vi "Pickering 4 wire.vi"(0 "26":string[](array[combo])=["y5"], 1 "27":string[](array[combo])=["NC"], 2 "28":string[](array[combo])=["y3"], 3 "1":string[](array[combo])=["y4", "NC"], 8 "5":string[](array[combo])=["NC"], 9 "4":string[](array[combo])=["y6"], 10 "3":string[](array[combo])=["NC"], 11 "2":string[](array[combo])=["y1"]) -> ()   [LabVIEW 2011]
panel:
  in  "Initialize":bool
  in  "Pickering status":path=path "C:/LabView/PPMS basic VIs/Switch Status.txt"
  in  "Disconnect all?":bool
  in  "IVI Option String":string="Simulate=0,RangeCheck=1,QueryInstrStatus=0,Cache=1,DriverSetup=Model:40-726-511-M;"
  in  "VISA Resource Name":string="PXI9::13::INSTR"
  in  "X Channel Ground":string="x12"
  in  "Discharge Y Channels?":bool=TRUE
  in  "Discharge X channels?":bool=TRUE
  in  "Y Channel Ground":string="y1"
  # "4 wire              measurements\nFeature:\n1, Multiple connections\n2, Make before break\n3, First run resets device\n\nNotes:\nLock-in 1: I+/I- -->AO0/AI0, board 0\n\nLock-in 3: V+/V-  --> AI0, board 1.  \n  V+/V- conencted to y3 and y4. OSC output should set the same as Lock-in 1\n\nLock-in 2: I2+/I2- -->AO1/AI1, board 0\n\nLock-in 4: V2+/V2- -> y7/y8"
  # "1"
  # "3"
  # "2"
  # "26"
  # "5"
  # "4"
  # "28"
  # "27"
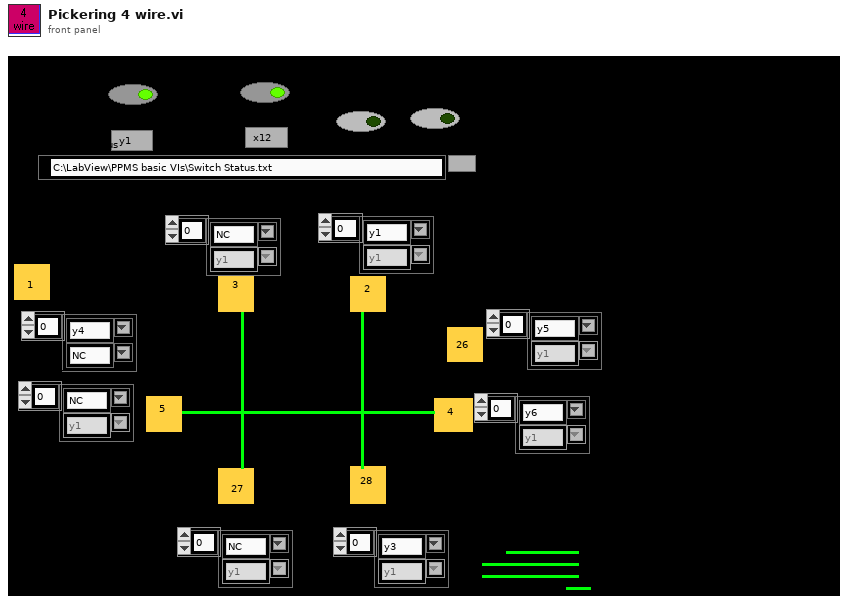
[diagram p1: front panel]
types:
  T1 = cluster{"output string":string, "output string":string}
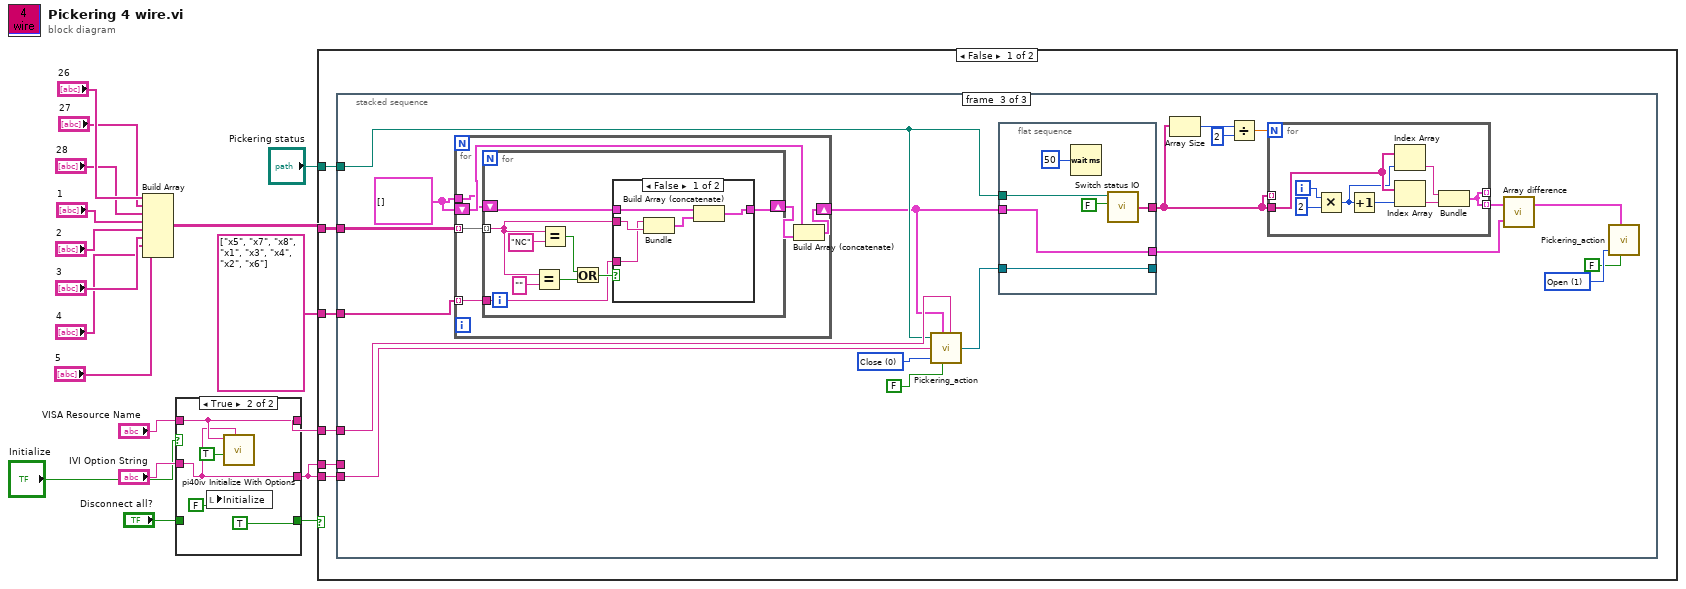
[diagram p0: block diagram]
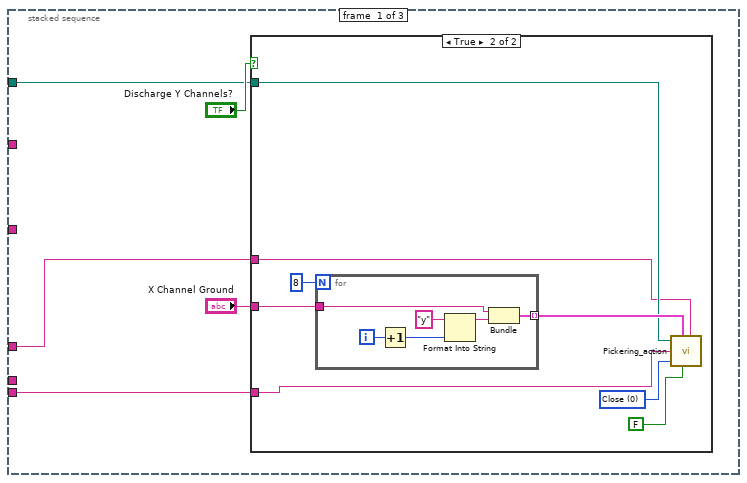
[diagram p3: hidden frame]
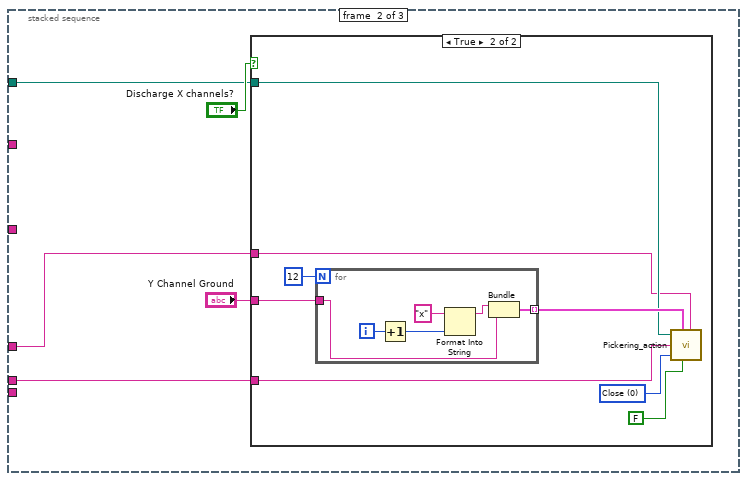
[diagram p5: hidden frame]
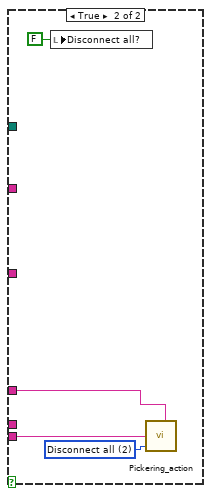
[diagram p8: hidden frame]
diagram:
  n1 = Build Array("26", "27", "28", "1", "2", "3", "4", "5") -> (w8:string[][])
  n2 = case shown="True" "Initialize" {
    tunnel: "VISA Resource Name" -> [w21 w26]
    tunnel: [w21 w26] -> w6
    tunnel: "IVI Option String" -> [w20 w25]
    tunnel: [w20 w25] -> w4
    tunnel: "Disconnect all?" -> [w19 _]
    tunnel: [w19 TRUE ("reset device")] -> w1
    frame False {
    }
    frame True {
      n3 = local write "Initialize"(FALSE ("reset device")) -> ()
      n4 = call <instrlib>:"pi40iv Initialize With Options.vi"("option string"=w25, "reset device"=TRUE, "resource name"=w26) -> ()  [unwired: 7 in, 2 out]
    }
  }
  n5 = case shown="False" w1 {
    tunnel: w8 -> [w32 _]
    tunnel: string[] ["x5", "x7", "x8", "x1", "x3", "x4", "x2", "x6"] -> [w31 _]
    tunnel: w4 -> [w30 w126]
    tunnel: w6 -> [w29 w125]
    tunnel: "Pickering status" -> [w28 _]
    tunnel: w4 -> [w27 _]
    frame False {
      n6 = stacked-sequence {
        tunnel: w32 -> [_ _ w89]
        tunnel: w31 -> [_ _ w88]
        tunnel: w30 -> [w35 _ w87]
        tunnel: w29 -> [w33 w53 w86]
        tunnel: w28 -> [w34 w54 w85]
        tunnel: w27 -> [_ w52 _]
        frame #0 {
          n7 = case shown="True" "Discharge Y Channels?" {
            tunnel: "X Channel Ground" -> [_ w45]
            tunnel: w35 -> [_ w41]
            tunnel: w33 -> [_ w38]
            tunnel: w34 -> [_ w40]
            frame False {
            }
            frame True {
              w42 = u16 0 items=["Close", "Open", "Disconnect all"] ("Action")
              n8 = for {
                N: 8 -> [_]
                tunnel: w45 -> [w47]
                tunnel: [w46] -> w43 mode=indexing
                i -> [w50]
                n9 = Increment(x=w50) -> (x+1=w49:i32)
                n10 = Format Into String(initial string="y", w49) -> (resulting string=w48:string)  [unwired: 2 in, 1 out]
                n11 = Bundle("X Channel Ground"=w47, w48) -> (w46:cluster{"X Channel Ground":string, string})  [unwired: 1 in]
              }
              n12 = call "Pickering_action.vi"("Pickering status"=w40, "Array"=w43, "option string"=w41, "Action"=w42, "Initialize"=FALSE, "resource name"=w38) -> ()  [unwired: 3 in, 1 out]
            }
          }
        }
        frame #1 {
          n13 = case shown="True" "Discharge X channels?" {
            tunnel: "Y Channel Ground" -> [_ w64]
            tunnel: w54 -> [_ w61]
            tunnel: w53 -> [_ w60]
            tunnel: w52 -> [_ w59]
            frame False {
            }
            frame True {
              w57 = u16 0 items=["Close", "Open", "Disconnect all"] ("Action")
              n14 = for {
                N: 12 -> [_]
                tunnel: w64 -> [w65]
                tunnel: [w67] -> w62 mode=indexing
                i -> [w69]
                n15 = Increment(x=w69) -> (x+1=w68:i32)
                n16 = Format Into String(initial string="x", w68) -> (resulting string=w66:string)  [unwired: 2 in, 1 out]
                n17 = Bundle(w66, "Y Channel Ground"=w65) -> (w67:cluster{string, "Y Channel Ground":string})  [unwired: 1 in]
              }
              n18 = call "Pickering_action.vi"("Pickering status"=w61, "Array"=w62, "option string"=w59, "Action"=w57, "Initialize"=FALSE, "resource name"=w60) -> ()  [unwired: 3 in, 1 out]
            }
          }
        }
        frame #2 {
          w76 = u16 1 items=["Close", "Open", "Disconnect all"] ("Action")
          w84 = u16 0 items=["Close", "Open", "Disconnect all"] ("Action")
          w80 = cluster{"5":string, string}[] []
          n19 = for {
            tunnel: w89 -> [w108] mode=indexing
            tunnel: w88 -> [w109] mode=indexing
            shift-right: [w107] -> w81
            shift-left: w80 -> [w105]
            tunnel: w80 -> [w104]
            n20 = for {
              tunnel: w109 -> [w113]
              tunnel: w108 -> [w112] mode=indexing
              shift-right: [w110] -> w106
              shift-left: w104 -> [w111]
              n21 = Equal?(x=w112, y="") -> (x = y?=w115:bool)
              n22 = Equal?(x=w112, y="NC") -> (x = y?=w117:bool)
              n23 = Or(x=w117, y=w115) -> (x .or. y?=w116:bool)
              n24 = case shown="False" w116 {
                tunnel: w113 -> [w119 _]
                tunnel: w112 -> [w120 _]
                tunnel: [w122 w124] -> w110
                tunnel: w111 -> [w121 w124]
                frame False {
                  n25 = Bundle(w119, "26"=w120) -> (w123:cluster{string, "26":string})  [unwired: 1 in]
                  n26 = Build Array (concatenate)(w121, w123) -> (w122:cluster{"5":string, "26":string}[])
                }
                frame True {
                }
              }
            }
            n27 = Build Array (concatenate)(w105, w106) -> (w107:cluster{"5":string, string}[])
          }
          n28 = call "Pickering_action.vi"("Pickering status"=w85, "Array"=w81, "option string"=w87, "Action"=w84, "Initialize"=FALSE, "resource name"=w86) -> ("instrument handle out"=w82:refnum<k15>)  [unwired: 3 in]
          n29 = flat-sequence {
            tunnel: w82 -> [w102]
            tunnel: [w102] -> _
            tunnel: [w101] -> w75
            tunnel: w85 -> [w100]
            tunnel: w81 -> [w98]
            tunnel: [w98] -> w73
            frame #0 {
              n30 = Wait (ms)(milliseconds to wait=u32 50) -> ()  [unwired: 1 out]
              n31 = call "Switch status IO.vi"("Write: T\nRead: F"=FALSE ("Write: T\nRead: F"), "Path"=w100) -> ("String out"=w101:string[])  [unwired: 4 in]
            }
          }
          n32 = Array Size(array=w75) -> (size(s)=w79:i32)
          n33 = Divide(x=w79, y=2) -> (x/y=w77:dbl)
          n34 = for {
            N: w77 -> [_]
            tunnel: w75 -> [w97]
            tunnel: w75 -> [_] mode=indexing
            tunnel: [w90] -> _ mode=indexing
            tunnel: [w90] -> w74 mode=indexing
            i -> [w93]
            n35 = Multiply(x=w93, y=2) -> (x*y=w91:i32)
            n36 = Increment(x=w91) -> (x+1=w96:i32)
            n37 = Index Array(array=w97, index=w91) -> (element=w95:string)
            n38 = Index Array(array=w97, index=w96) -> (element=w94:string)
            n39 = Bundle("output string"=w95, "output string"=w94) -> (w90:T1)  [unwired: 1 in]
          }
          n40 = call "Array difference.vi"("Array 2"=w73, "Array 1"=w74) -> ("Array 1-(array1&2)"=w72:cluster{"String":string, "String 2":string}[])  [unwired: 1 out]
          n41 = call "Pickering_action.vi"("Array"=w72, "Action"=w76, "Initialize"=FALSE) -> ()  [unwired: 6 in, 1 out]
        }
      }
    }
    frame True {
      w127 = u16 2 items=["Close", "Open", "Disconnect all"] ("Action")
      n42 = local write "Disconnect all?"(FALSE ("Disconnect all?")) -> ()
      n43 = call "Pickering_action.vi"("option string"=w126, "Action"=w127, "resource name"=w125) -> ()  [unwired: 6 in, 1 out]
    }
  }
